vi "Limelight Alignment.vi"(0 "Turn On?":bool, 1 "Drive Ref":string) -> ()   [LabVIEW 2018]
uses:
  <vilib>/Rock Robotics/WPI/Utilities/WPI_GetSetVariantRefNum.vi
  <vilib>/Rock Robotics/Network Tables/NT Read Number.vi
  <vilib>/Rock Robotics/WPI/RobotDrive/WPI_RobotDriveArcadeDrive_Standard(NoSaturation).vi
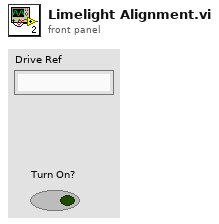
[diagram p1: front panel]
types:
  T1 = typedef "WPI_RobotDriveDevRef.ctl" = cluster{"DevStatus":errorcluster, "Motors[]":T2[], "Square Inputs":bool, "Max Output":dbl}
  T2 = typedef "WPI_MotorControlDeviceRef.ctl" = cluster{"DeviceStatus":errorcluster, "Type":T3, "PWM":cluster{"PWM Channel":T4, "DeadBand":T5}, "CAN":cluster{"Device Number":u8, "SetOutput VI Ref":variant, "GetOutput VI Ref":variant, "Enable VI Ref":variant, "Disable VI Ref":variant, "Data":variant}, "Invert":bool, "DIO PWM":cluster{"PWM \"Enable\" Channel":T4, "DIOChannel":T6, "PWM Rate":dbl}}
  T3 = typedef "WPI_MotorControlType.ctl" = enum16{"PWM", "CAN", "DIO PWM"}
  T4 = typedef "FPGA_DIOPWMChannel.ctl" = enum8{"PWM 0", "PWM 1", "PWM 2", "PWM 3", "PWM 4", "PWM 5", "PWM 6", "PWM 7", "PWM 8", "PWM 9", "PWM MXP 0", "PWM MXP 1", "PWM MXP 2", "PWM MXP 3", "PWM MXP 4", "PWM MXP 5", "PWM MXP 6", "PWM MXP 7", "PWM MXP 8", "PWM MXP 9", "Invalid"}
  T5 = typedef "WPI_PWMDeadband.ctl" = cluster{"Name":string, "maxPositivePwm":i32, "minPositivePwm":i32, "centerPwm":i32, "maxNegativePwm":i32, "minNegativePwm":i32, "angularRange":u16}
  T6 = typedef "FPGA_DIOChannel.ctl" = enum8{"DIO 0", "DIO 1", "DIO 2", "DIO 3", "DIO 4", "DIO 5", "DIO 6", "DIO 7", "DIO 8", "DIO 9", "DIO MXP 0", "DIO MXP 1", "DIO MXP 2", "DIO MXP 3", "DIO MXP 4", "DIO MXP 5", "DIO MXP 6", "DIO MXP 7", "DIO MXP 8", "DIO MXP 9", "DIO MXP 10", "DIO MXP 11", "DIO MXP 12", "DIO MXP 13", "DIO MXP 14", "DIO MXP 15", "SPI Port CS1", "SPI Port CS2", "SPI Port CS3", "SPI Port MISO", "SPI Port MOSI", "Invalid"}
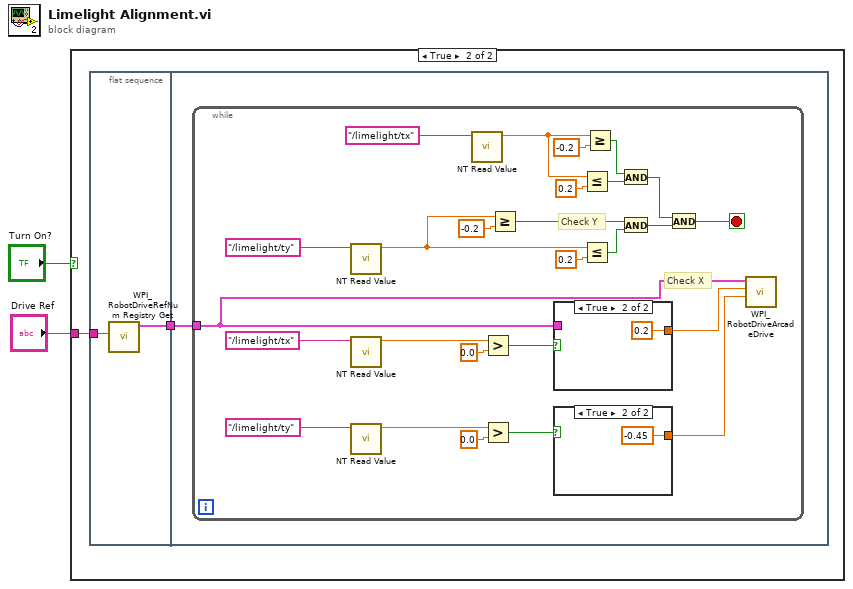
[diagram p0: block diagram]
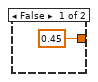
[diagram p3: hidden frame]
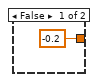
[diagram p4: hidden frame]
diagram:
  n1 = case shown="True" "Turn On?" {
    tunnel: "Drive Ref" -> [_ w4]
    frame False {
    }
    frame True {
      n2 = flat-sequence {
        tunnel: w4 -> [w6]
        tunnel: [w5] -> w3
        tunnel: w3 -> [w7]
        frame #0 {
          n3 = call <vilib>:"WPI_RobotDriveRefNum Registry Get.vi"("refnum name"=w6) -> ("RobotDriveDevRef"=w5:T1)  [unwired: 9 in, 1 out]
        }
        frame #1 {
          n4 = while {
            tunnel: w7 -> [w14]
            stop <- w23 stop-if-true
            # "Check Y"
            # "Check X"
            n5 = call-poly <vilib>:"NT Read Value.vi"("Name"="/limelight/ty") -> ("Numeric"=w19:dbl)  [unwired: 9 in, 1 out]
            n6 = call-poly <vilib>:"NT Read Value.vi"("Name"="/limelight/tx") -> ("Numeric"=w16:dbl)  [unwired: 9 in, 1 out]
            n7 = call-poly <vilib>:"NT Read Value.vi"("Name"="/limelight/ty") -> ("Numeric"=w12:dbl)  [unwired: 9 in, 1 out]
            n8 = call-poly <vilib>:"NT Read Value.vi"("Name"="/limelight/tx") -> ("Numeric"=w21:dbl)  [unwired: 9 in, 1 out]
            n9 = Greater?(x=w16, y=0.0) -> (0:w18:bool)
            n10 = Greater?(x=w12, y=0.0) -> (0:w10:bool)
            n11 = Greater Or Equal?(x=w19, y=-0.2) -> (x >= y?=w33:bool)
            n12 = case shown="True" w18 {
              tunnel: w14 -> [_ _]
              tunnel: [-0.2 0.2] -> w8
              frame False {
              }
              frame True {
              }
            }
            n13 = case shown="True" w10 {
              tunnel: [0.45 -0.45] -> w9
              frame False {
              }
              frame True {
              }
            }
            n14 = Less Or Equal?(x=w21, y=0.2) -> (x <= y?=w27:bool)
            n15 = Less Or Equal?(x=w19, y=0.2) -> (x <= y?=w32:bool)
            n16 = Greater Or Equal?(x=w21, y=-0.2) -> (x >= y?=w26:bool)
            n17 = And(x=w26, y=w27) -> (x .and. y?=w25:bool)
            n18 = And(x=w33, y=w32) -> (x .and. y?=w24:bool)
            n19 = And(x=w25, y=w24) -> (x .and. y?=w23:bool)
            n20 = call-poly <vilib>:"WPI_RobotDriveArcadeDrive.vi"("Y axis value"=w9, "X axis value"=w8, "RobotDriveDevRef"=w14) -> ()  [unwired: 6 in, 3 out]
          }
        }
      }
    }
  }
